vi "Post-Build Action_for_Overlays.vi"(5 "Files Generated by Build":path[](array[path]), 6 "Top Level/Always Included VIs":path[](array[path]), 7 "Destination Path":path, 8 "error in (no error)":errorcluster, 9 "Target Name":string, 10 "Build Specification Name":string, 11 "Project Path":path) -> (0 "error out":errorcluster)   [LabVIEW 2018]
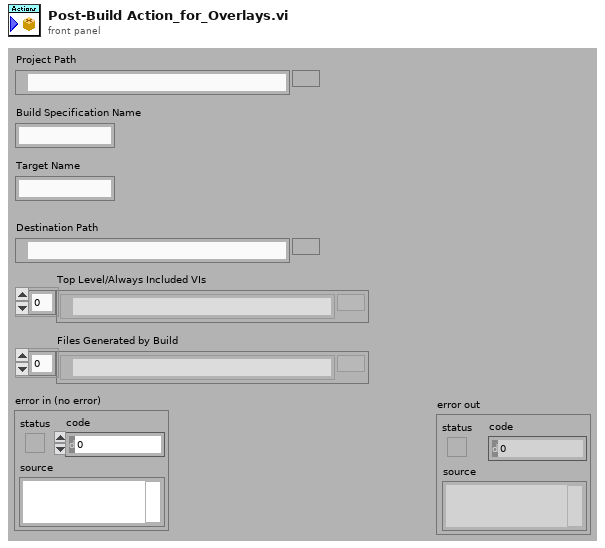
[diagram p1: front panel]
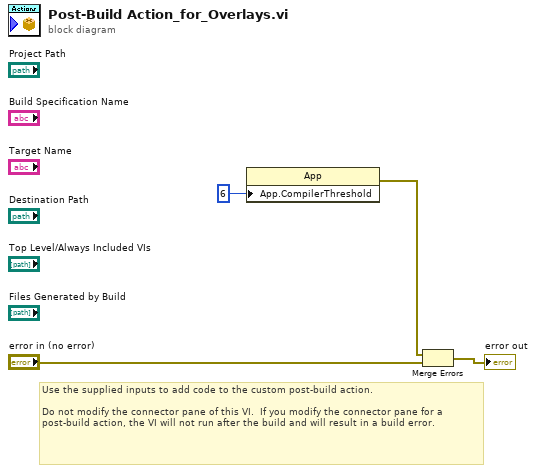
[diagram p0: block diagram]
diagram:
  # "Use the supplied inputs to add code to the custom post-build action.\n\nDo not modify the connector pane of this VI.  If you modify the connector pane for a post-build action, the VI will not run after the build and will result in a build error."
  n1 = property class="App"("App.CompilerThreshold"=u32 6 ("Application:Compiler Threshold")) -> (error out=w1:errorcluster)  [unwired: 2 in, 1 out]
  n2 = Merge Errors(w1, "error in (no error)") -> (→"error out":errorcluster)
